vi "ZMQ Req Test.vi"() -> ()   [LabVIEW 2019, in "RemoteControl.ZMQ.lvlib" / "RemoteControl.ZMQ.lvclass"]
uses:
  RemoteControl.ZMQ.lvclass
  <vilib>/addons/zeromq/zmq_context.lvclass
  <vilib>/addons/zeromq/zmq_socket.lvclass
  <vilib>/addons/zeromq/socket_type.ctl
  <vilib>/addons/zeromq/zeromq.lvlib
  <vilib>/addons/zeromq/socket_options.ctl
  <userlib>/LevyLab/RemoteControl/RemoteControl/RemoteControl.lvclass
  C:/Program Files (x86)/National Instruments/LabVIEW 2019/user.lib/LevyLab/RemoteControl/RemoteControl/RemoteControl.lvclass
  C:/Program Files (x86)/National Instruments/LabVIEW 2019/vi.lib/JKI/JKI SMO/smo.lvlibp/SMO/SMO.lvclass
panel:
  in  "milliseconds to wait":u32
  out "msg/s":dbl
  in  "stop":bool
  out "Data out":variant
  out "error out":errorcluster
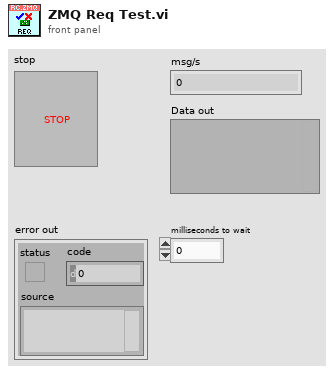
[diagram p1: front panel]
types:
  T1 = typedef "zeromq.lvlib/socket_options.ctl" = enum8{"NONE", "ZMQ_HWM", "<2>", "ZMQ_SWAP", "ZMQ_AFFINITY", "ZMQ_ROUTING_ID", "ZMQ_SUBSCRIBE", "ZMQ_UNSUBSCRIBE", "ZMQ_RATE", "ZMQ_RECOVERY_IVL", "ZMQ_MCAST_LOOP", "ZMQ_SNDBUF", "ZMQ_RCVBUF", "ZMQ_RCVMORE", "ZMQ_FD", "ZMQ_EVENTS", "ZMQ_TYPE", "ZMQ_LINGER", "ZMQ_RECONNECT_IVL", "ZMQ_BACKLOG", "ZMQ_RECOVERY_IVL_MSEC", "ZMQ_RECONNECT_IVL_MAX", "ZMQ_MAXMSGSIZE", "ZMQ_SNDHWM", "ZMQ_RCVHWM", "ZMQ_MULTICAST_HOPS", "<26>", "ZMQ_RCVTIMEO", "ZMQ_SNDTIMEO", "<29>", "<30>", "ZMQ_IPV4ONLY", "ZMQ_LAST_ENDPOINT", "ZMQ_ROUTER_MANDATORY", "ZMQ_TCP_KEEPALIVE", "ZMQ_TCP_KEEPALIVE_CNT", "ZMQ_TCP_KEEPALIVE_IDLE", "ZMQ_TCP_KEEPALIVE_INTVL", "ZMQ_TCP_ACCEPT_FILTER", "ZMQ_IMMEDIATE", "ZMQ_XPUB_VERBOSE", "ZMQ_ROUTER_RAW", "ZMQ_IPV6", "ZMQ_MECHANISM", "ZMQ_PLAIN_SERVER", "ZMQ_PLAIN_USERNAME", "ZMQ_PLAIN_PASSWORD", "ZMQ_CURVE_SERVER", "ZMQ_CURVE_PUBLICKEY", "ZMQ_CURVE_SECRETKEY", "ZMQ_CURVE_SERVERKEY", "ZMQ_PROBE_ROUTER", "ZMQ_REQ_CORRELATE", "ZMQ_REQ_RELAXED", "ZMQ_CONFLATE", "ZMQ_ZAP_DOMAIN", "ZMQ_ROUTER_HANDOVER", "ZMQ_TOS", "ZMQ_IPC_FILTER_PID", "ZMQ_IPC_FILTER_UID", "ZMQ_IPC_FILTER_GID", "ZMQ_CONNECT_ROUTING_ID", "ZMQ_GSSAPI_SERVER", "ZMQ_GSSAPI_PRINCIPAL", "ZMQ_GSSAPI_SERVICE_PRINCIPAL", "ZMQ_GSSAPI_PLAINTEXT", "ZMQ_HANDSHAKE_IVL", "<67>", "ZMQ_SOCKS_PROXY", "ZMQ_XPUB_NODROP", "ZMQ_BLOCKY", "ZMQ_XPUB_MANUAL", "ZMQ_XPUB_WELCOME_MSG", "ZMQ_STREAM_NOTIFY", "ZMQ_INVERT_MATCHING", "ZMQ_HEARTBEAT_IVL", "ZMQ_HEARTBEAT_TTL", "ZMQ_HEARTBEAT_TIMEOUT", "ZMQ_XPUB_VERBOSER", "ZMQ_CONNECT_TIMEOUT", "ZMQ_TCP_MAXRT", "ZMQ_THREAD_SAFE", "<82>", "<83>", "ZMQ_MULTICAST_MAXTPDU", "ZMQ_VMCI_BUFFER_SIZE", "ZMQ_VMCI_BUFFER_MIN_SIZE", "ZMQ_VMCI_BUFFER_MAX_SIZE", "ZMQ_VMCI_CONNECT_TIMEOUT", "ZMQ_USE_FD", "ZMQ_GSSAPI_PRINCIPAL_NAMETYPE", "ZMQ_GSSAPI_SERVICE_PRINCIPAL_NAMETYPE", "ZMQ_BINDTODEVICE", "ZMQ_ZAP_ENFORCE_DOMAIN", "ZMQ_LOOPBACK_FASTPATH", "ZMQ_METADATA", "ZMQ_MULTICAST_LOOP", "ZMQ_ROUTER_NOTIFY"}
  T2 = typedef "zeromq.lvlib/socket_type.ctl" = enum8{"ZMQ_PAIR", "ZMQ_PUB", "ZMQ_SUB", "ZMQ_REQ", "ZMQ_REP", "ZMQ_DEALER", "ZMQ_ROUTER", "ZMQ_PULL", "ZMQ_PUSH", "ZMQ_XPUB", "ZMQ_XSUB", "ZMQ_STREAM", "ZMQ_SERVER", "ZMQ_CLIENT", "ZMQ_RADIO", "ZMQ_DISH", "ZMQ_GATHER", "ZMQ_SCATTER", "ZMQ_DGRAM"}
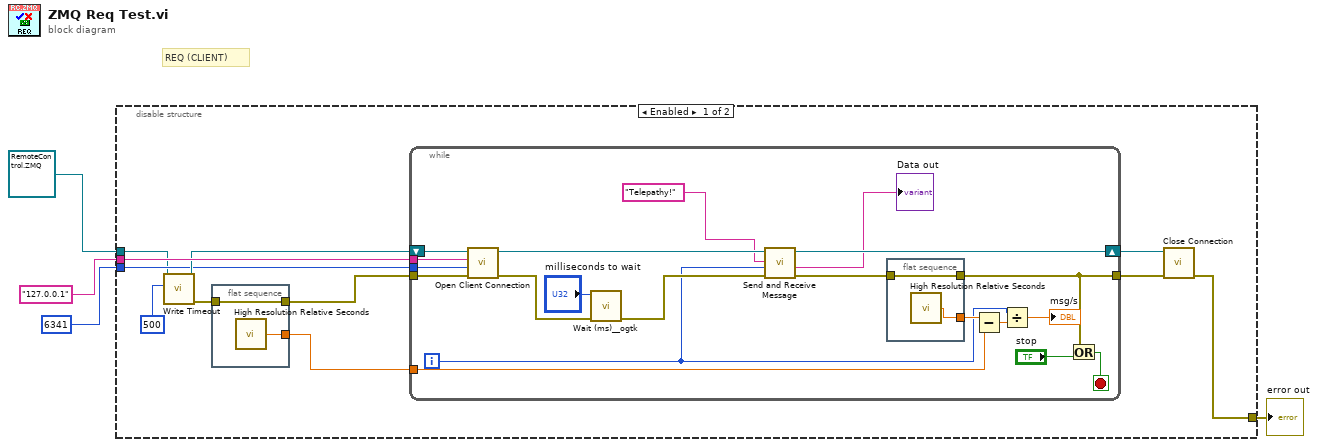
[diagram p0: block diagram]
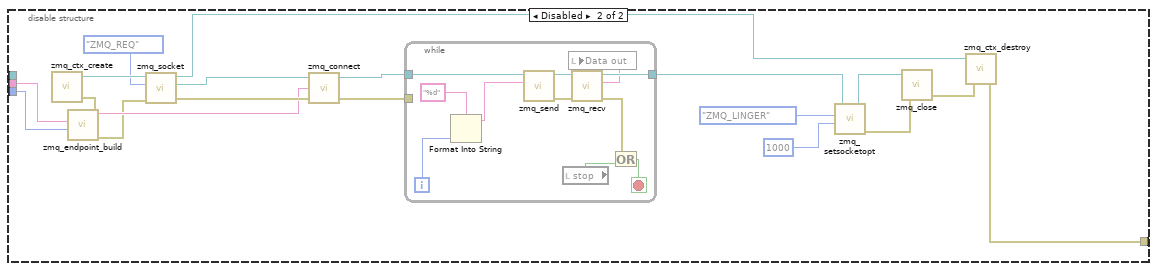
[diagram p2: hidden frame]
diagram:
  # "REQ (CLIENT)"
  n1 = disable-structure shown="Enabled" {
    disable-tunnel: [w13 w41] -> w4
    disable-tunnel: "127.0.0.1" ("Address") -> [w11 w52]
    disable-tunnel: u16 6341 ("Port") -> [w9 w53]
    disable-tunnel: refnum<class "RemoteControl.ZMQ.lvclass"> refnum ("RemoteControl.ZMQ.lvlib:RemoteControl.ZMQ.lvclass") -> [w5 _]
    frame Enabled {
      n2 = call <userlib>:"Write Timeout.vi"("timeout (ms) [500]"=500 ("timeout in ms (100)"), "RemoteControl in"=w5) -> ("error out"=w8:errorcluster, "RemoteControl out"=w10:refnum<class "RemoteControl.ZMQ.lvclass">)  [unwired: 8 in]
      n3 = flat-sequence {
        tunnel: [w17] -> w6
        tunnel: w8 -> [w17]
        tunnel: [w16] -> w7
        frame #0 {
          n4 = call <vilib>:"High Resolution Relative Seconds.vi"() -> ("relative seconds"=w16:dbl)
        }
      }
      n5 = while {
        tunnel: [w28] -> w14
        tunnel: w6 -> [w26]
        tunnel: w7 -> [w31]
        shift-right: [w37] -> w15
        shift-left: w10 -> [w27]
        tunnel: w9 -> [w25]
        tunnel: w11 -> [w24]
        i -> [w19]
        stop <- w33 stop-if-true
        n6 = call-dynamic "Open Client Connection.vi"("error in (no error)"=w26, "Port"=w25, "address"=w24, "RemoteControl.ZMQ in"=w27) -> ("error out"=w22:errorcluster, "RemoteControl.ZMQ out"=w20:refnum<class "RemoteControl.ZMQ.lvclass">)  [unwired: 6 in]
        n7 = call <userlib>:"Wait (ms)__ogtk.vi"("error in (no error)"=w22, "milliseconds to wait"="milliseconds to wait") -> ("error out"=w21:errorcluster)  [unwired: 8 in, 1 out]
        n8 = call-dynamic "Send and Receive Message.vi"("error in (no error)"=w21, "Data"=w19, "Command"="Telepathy!", "RemoteControl in"=w20) -> ("error out"=w34:errorcluster, "Data out"=→"Data out":string, "RemoteControl out"=w37:refnum<class "RemoteControl.ZMQ.lvclass">)  [unwired: 4 in, 1 out]
        n9 = flat-sequence {
          tunnel: [w39] -> w28
          tunnel: w34 -> [w39]
          tunnel: [w38] -> w32
          frame #0 {
            n10 = call <vilib>:"High Resolution Relative Seconds.vi"() -> ("relative seconds"=w38:dbl)
          }
        }
        n11 = Subtract(x=w32, y=w31) -> (x-y=w30:dbl)
        n12 = Divide(x=w19, y=w30) -> (x/y=→"msg/s":dbl)
        n13 = Or(x=w28, y="stop") -> (x .or. y?=w33:bool)
      }
      n14 = call-dynamic "Close Connection.vi"("error in (no error)"=w14, "RemoteControl.ZMQ in"=w15) -> ("error out"=w13:errorcluster)  [unwired: 8 in, 1 out]
    }
    frame Disabled {
      n15 = call <vilib>:"zmq_ctx_create.vi"() -> ("error out"=w49:errorcluster, "context out"=w56:refnum<class "zmq_context.lvclass">)  [unwired: 4 in]
      n16 = call <vilib>:"zmq_endpoint_build.vi"("error in"=w49, "port"=w53, "address"=w52) -> ("error out"=w48:errorcluster, "endpoint"=w54:string)  [unwired: 2 in, 1 out]
      n17 = call <vilib>:"zmq_socket.vi"("error in"=w48, "socket type"=socket_type."ZMQ_REQ", "context in"=w56) -> ("error out"=w58:errorcluster, "socket out"=w57:refnum<class "zmq_socket.lvclass">, "context out"=w42:refnum<class "zmq_context.lvclass">)  [unwired: 2 in]
      n18 = call <vilib>:"zmq_connect.vi"("error in"=w58, "endpoint"=w54, "socket in"=w57) -> ("error out"=w51:errorcluster, "socket out"=w50:refnum<class "zmq_socket.lvclass">)  [unwired: 1 in]
      n19 = while {
        tunnel: w51 -> [_]
        tunnel: w50 -> [w69]
        tunnel: [w62] -> w45
        i -> [w65]
        stop <- w63 stop-if-true
        n20 = Format Into String(format string="%d" ("Command"), w65) -> (resulting string=w59:string)  [unwired: 2 in, 1 out]
        n21 = call <vilib>:"zmq_send.vi"("data"=w59, "socket in"=w69) -> ("error out"=w68:errorcluster, "socket out"=w67:refnum<class "zmq_socket.lvclass">)  [unwired: 5 in]
        n22 = local read "stop"() -> (w64:bool)
        n23 = call <vilib>:"zmq_recv.vi"("error in"=w68, "socket in"=w67) -> ("error out"=w60:errorcluster, "data"=w61:string, "socket out"=w62:refnum<class "zmq_socket.lvclass">)  [unwired: 3 in, 2 out]
        n24 = local write "Data out"(w61) -> ()
        n25 = Or(x=w60, y=w64) -> (x .or. y?=w63:bool)
      }
      n26 = call <vilib>:"zmq_setsocketopt.vi"("value"=1000, "option"=socket_options."ZMQ_LINGER", "socket in"=w45) -> ("error out"=w44:errorcluster, "socket out"=w46:refnum<class "zmq_socket.lvclass">)  [unwired: 3 in]
      n27 = call <vilib>:"zmq_close.vi"("error in"=w44, "socket"=w46) -> ("error out"=w43:errorcluster)  [unwired: 3 in]
      n28 = call <vilib>:"zmq_ctx_destroy.vi"("error in"=w43, "context in"=w42) -> ("error out"=w41:errorcluster)  [unwired: 3 in]
    }
  }
  "error out" <- w4
